vi "WaitAnswer.vi"(0 "VISA resource name out":refnum<visa-resource-name>) -> ()   [LabVIEW 2016]
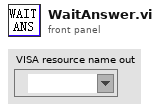
[diagram p1: front panel]
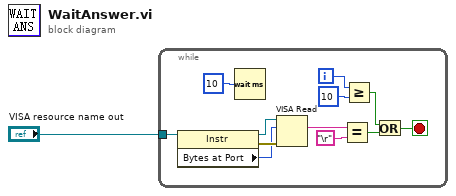
[diagram p0: block diagram]
diagram:
  n1 = while {
    tunnel: "VISA resource name out" -> [w8]
    i -> [w12]
    stop <- w6 stop-if-true
    n2 = property class="Instr"(reference=w8) -> (reference out=w10:refnum<visa-resource-name>, error out=w9:errorcluster, "Bytes at Port"=w7:u32)  [unwired: 1 in]
    n3 = Wait (ms)(milliseconds to wait=u32 10 ("等待时间（毫秒）")) -> ()  [unwired: 1 out]
    n4 = VISA Read(VISA resource name=w10, byte count=w7, error in (no error)=w9) -> (read buffer=w5:string)  [unwired: 3 out]
    n5 = Equal?(x=w5, y="\r") -> (x = y?=w2:bool)
    n6 = Greater Or Equal?(x=w12, y=10) -> (x >= y?=w3:bool)
    n7 = Or(x=w3, y=w2) -> (x .or. y?=w6:bool)
  }
